vi "fields new or copy field.vi"(4 "error in (no error)":errorcluster, 5 "All Fields (empty)":T1[](array[typedef]), 7 "Copy Existing? (\"\": new field)":string) -> (0 "error out":errorcluster, 1 "New Field Record":T1={"ixField"=0, "iSequenceOrder"=0, "sxFieldId"="", "sxSequenceId"="", "sDisplayName"="", "sValue"="", "sUnits"="", "nDataType"=enum."timestamp", "nNextItem"=enum."Reset", "fSystem"=FALSE, "fSystemValue"=FALSE, "fRequired"=FALSE, "fSetAtTest"=FALSE, "fTestField"=FALSE, "fDeleted"=FALSE, "fIndexed"=FALSE, "fFreeList"=FALSE})   [LabVIEW 2011]
uses:
  server/database/Fields/Field Record.ctl
  server/database/Fields/Field DataTypes.ctl
  server/database/Fields/Field NextItem.ctl
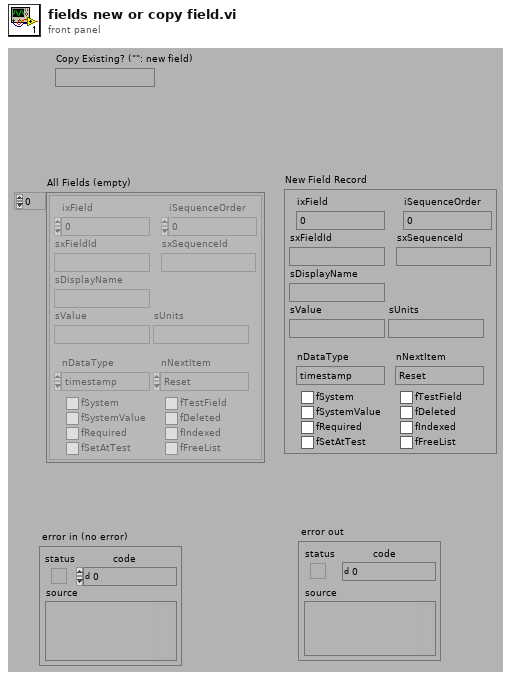
[diagram p1: front panel]
types:
  T1 = typedef "Field Record.ctl" = cluster{"ixField":i32, "iSequenceOrder":i32, "sxFieldId":string, "sxSequenceId":string, "sDisplayName":string, "sValue":string, "sUnits":string, "nDataType":T2, "nNextItem":T3, "fSystem":bool, "fSystemValue":bool, "fRequired":bool, "fSetAtTest":bool, "fTestField":bool, "fDeleted":bool, "fIndexed":bool, "fFreeList":bool}
  T2 = typedef "Field DataTypes.ctl" = enum32{"text", "numeric", "list", "timestamp", "boolean"}
  T3 = typedef "Field NextItem.ctl" = enum32{"Reset", "Retain", "Auto-Increment"}
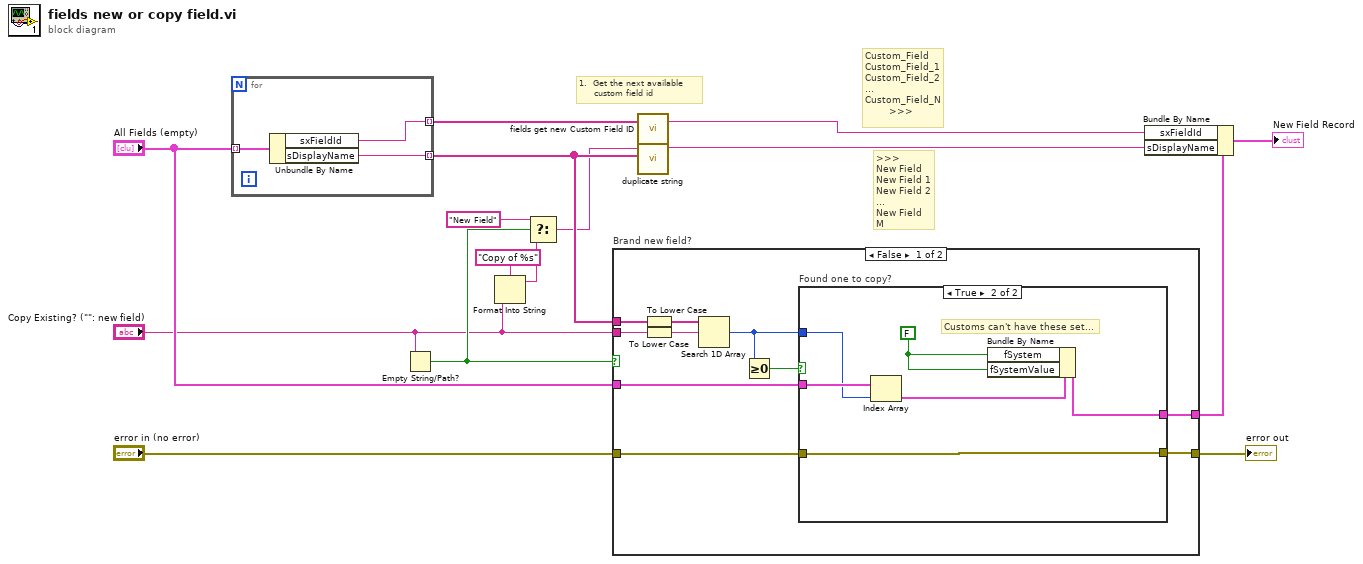
[diagram p0: block diagram]
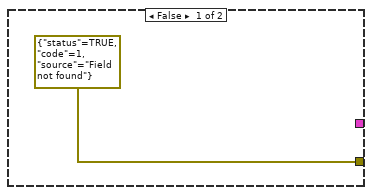
[diagram p2: hidden frame]
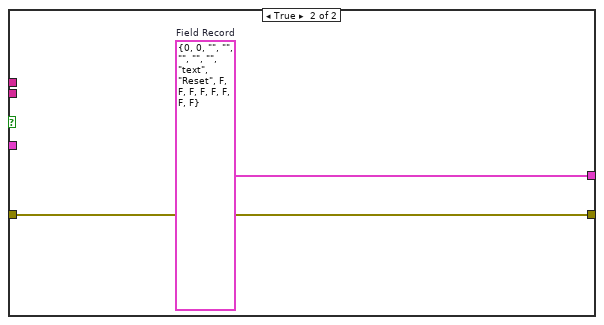
[diagram p3: hidden frame]
diagram:
  # ">>>\nNew Field\nNew Field 1\nNew Field 2\n...\nNew Field M"
  # "Custom_Field\nCustom_Field_1\nCustom_Field_2\n...\nCustom_Field_N\n        >>>"
  # "1.  Get the next available\n     custom field id"
  n1 = for {
    tunnel: "All Fields (empty)" -> [w18] mode=indexing
    tunnel: [w16] -> w2 mode=indexing
    tunnel: [w17] -> w9 mode=indexing
    n2 = Unbundle By Name(w18) -> ("sxFieldId"=w16:string, "sDisplayName"=w17:string)
  }
  n3 = Empty String/Path?(string/path="Copy Existing? (\"\": new field)") -> (empty?=w8:bool)
  n4 = Format Into String(format string="Copy of %s", "Copy Existing? (\"\": new field)") -> (resulting string=w4:string)  [unwired: 2 in, 1 out]
  n5 = Select(t="New Field" ("Desired Display Name (\"New Field\")"), s=w8, f=w4) -> (s? t:f=w7:string)
  n6 = case "Brand new field?" shown="False" w8 {
    tunnel: [w21 w37] -> w15
    tunnel: "Copy Existing? (\"\": new field)" -> [w26 _]
    tunnel: "error in (no error)" -> [w20 w36]
    tunnel: [w19 w36] -> w11
    tunnel: w9 -> [w28 _]
    tunnel: "All Fields (empty)" -> [w22 _]
    frame False {
      n7 = To Lower Case(string=w28) -> (all lower case string=w27:string[])
      n8 = To Lower Case(string=w26) -> (all lower case string=w25:string)
      n9 = Search 1D Array(1D array=w27, element=w25) -> (index of element=w23:i32)  [unwired: 1 out]
      n10 = Greater Or Equal To 0?(x=w23) -> (x >= 0?=w24:bool)
      n11 = case "Found one to copy?" shown="True" w24 {
        tunnel: w23 -> [_ w34]
        tunnel: w22 -> [_ w35]
        tunnel: [_ w31] -> w21
        tunnel: [errorcluster {"status"=TRUE, "code"=1, "source"="Field not found"} ("error in (no error)") w33] -> w19
        tunnel: w20 -> [_ w33]
        frame False {
        }
        frame True {
          w30 = FALSE
          # "Customs can't have these set..."
          n12 = Index Array(array=w35, index=w34) -> (element=w32:T1)
          n13 = Bundle By Name(cluster=w32, "fSystem"=w30, "fSystemValue"=w30) -> (w31:T1)
        }
      }
    }
    frame True {
      w37 = T1 {"ixField"=0, "iSequenceOrder"=0, "sxFieldId"="", "sxSequenceId"="", "sDisplayName"="", "sValue"="", "sUnits"="", "nDataType"=enum."text", "nNextItem"=enum."Reset", "fSystem"=FALSE, "fSystemValue"=FALSE, "fRequired"=FALSE, "fSetAtTest"=FALSE, "fTestField"=FALSE, "fDeleted"=FALSE, "fIndexed"=FALSE, "fFreeList"=FALSE}  # Field Record
    }
  }
  "error out" <- w11
  n14 = call "fields get new Custom Field ID.vi"("Existing Field IDs (empty)"=w2) -> ("Custom Field ID"=w1:string)  [unwired: 1 in, 1 out]
  n15 = call "duplicate string.vi"("Array of Strings"=w9, "String"=w7) -> ("Updated String"=w14:string)  [unwired: 9 out]
  n16 = Bundle By Name(cluster=w15, "sxFieldId"=w1, "sDisplayName"=w14) -> (→"New Field Record":T1)
